vi "02 Temperatura Final.vi"() -> ()   [LabVIEW 2021]
panel:
  out "Temperatura\nFinal":dbl(slide) scale=0.0..50.0
  in  "Calor":dbl
  in  "Temperatura\nInicial":dbl(slide) scale=0.0..50.0
  in  "Cantidad":dbl
  in  "Sustancia":dbl(ring)=2.4 items=["Alcohol Etílico"=2.4, "Agua"=4.186, "Glicerina"=2.43, "Benceno"=1.1881]
  in  "Unidades":dbl(ring) items=["Mol", "Kilogramo", "Litro"]
  in  "stop":bool
  # "TEMPERATURA FINAL"
  # "CONDICIONES"
  # "Desarrollado por:\n     Semillero Electroquimica e Innovación Ambiental - SEIA"
  # "°C"
  # "kJ"
  # "°C"
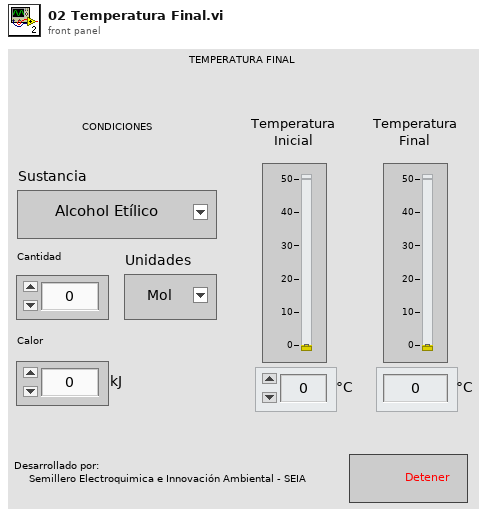
[diagram p1: front panel]
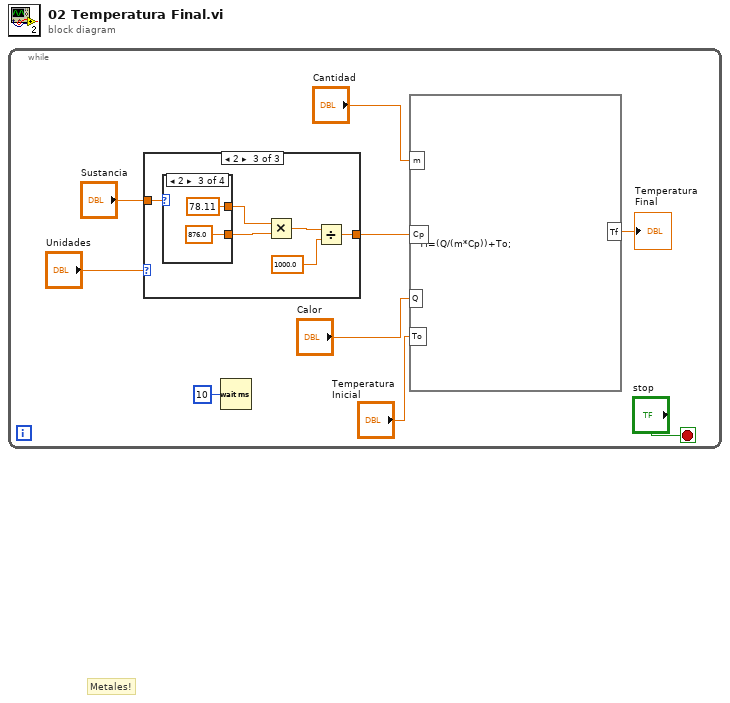
[diagram p0: block diagram]
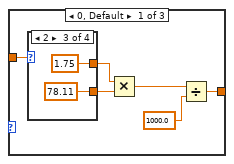
[diagram p2: hidden frame]
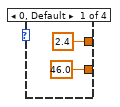
[diagram p3: hidden frame]
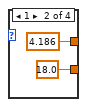
[diagram p4: hidden frame]
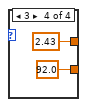
[diagram p5: hidden frame]
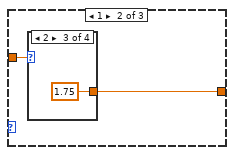
[diagram p6: hidden frame]
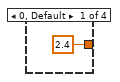
[diagram p7: hidden frame]
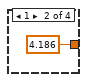
[diagram p8: hidden frame]
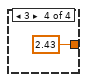
[diagram p9: hidden frame]
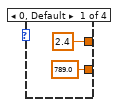
[diagram p10: hidden frame]
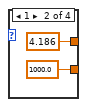
[diagram p11: hidden frame]
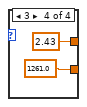
[diagram p12: hidden frame]
diagram:
  # "Metales!"
  n1 = while {
    stop <- "stop" stop-if-true
    n2 = case shown="2" "Unidades" {
      tunnel: "Sustancia" -> [w15 w25 w32]
      tunnel: [w12 w24 w30] -> w4
      frame 0, Default {
        n3 = case shown="2" w15 {
          tunnel: [2.4 4.186 1.75 2.43] -> w11
          tunnel: [46.0 18.0 78.11 92.0] -> w10
          frame 0, Default {
          }
          frame 1 {
          }
          frame 2 {
          }
          frame 3 {
          }
        }
        n4 = Multiply(x=w11, y=w10) -> (x*y=w14:dbl)
        n5 = Divide(x=w14, y=1000.0) -> (x/y=w12:dbl)
      }
      frame 1 {
        n6 = case shown="2" w25 {
          tunnel: [2.4 4.186 1.75 2.43] -> w24
          frame 0, Default {
          }
          frame 1 {
          }
          frame 2 {
          }
          frame 3 {
          }
        }
      }
      frame 2 {
        n7 = case shown="2" w32 {
          tunnel: [2.4 4.186 78.11 2.43] -> w34
          tunnel: [789.0 1000.0 876.0 1261.0] -> w31
          frame 0, Default {
          }
          frame 1 {
          }
          frame 2 {
          }
          frame 3 {
          }
        }
        n8 = Multiply(x=w34, y=w31) -> (x*y=w35:dbl)
        n9 = Divide(x=w35, y=1000.0) -> (x/y=w30:dbl)
      }
    }
    n10 = Wait (ms)(milliseconds to wait=u32 10) -> ()  [unwired: 1 out]
    n11 = formula code="Tf=(Q/(m*Cp))+To;"("Cp"=w4, "Q"="Calor", "To"="Temperatura\nInicial", "m"="Cantidad") -> ("Tf"=→"Temperatura\nFinal":dbl)
  }
